vi "IsInstanceOf.vi"(2 "is object instance of":refnum<class>, 3 "reference in":refnum<class "G#Object.lvclass">) -> (0 "is instance of":bool, 1 "reference out":refnum<class "G#Object.lvclass">)   [LabVIEW 2020, in "G#Object.lvclass"]
doc: "Checks if the input 'reference in' is of the same class or a subclass of the input 'is object instance of'."
uses:
  G#Object.lvclass
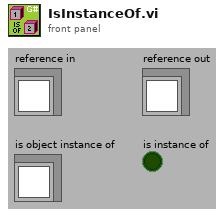
[diagram p1: front panel]
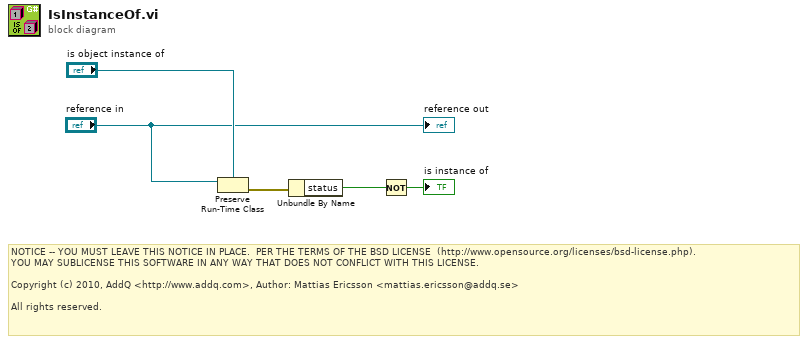
[diagram p0: block diagram]
diagram:
  # "NOTICE -- YOU MUST LEAVE THIS NOTICE IN PLACE.  PER THE TERMS OF THE BSD LICENSE  (http://www.opensource.org/licenses/bsd-license.php).\nYOU MAY SUBLICENSE THIS SOFTWARE IN ANY WAY THAT DOES NOT CONFLICT WITH THIS LICENSE.\n\nCopyright (c) 2010, AddQ <http://www.addq.com>, Author: Mattias Ericsson <mattias.ericsson@addq.se>\n\nAll rights reserved."
  n1 = Preserve Run-Time Class(object in="reference in", 2:"is object instance of") -> (error out=w2:errorcluster)  [unwired: 1 in, 1 out]
  n2 = Unbundle By Name(w2) -> ("status"=w1:bool)
  n3 = Not(x=w1) -> (.not. x?=→"is instance of":bool)
  "reference out" <- "reference in"
